vi "Analogico_digital_Controlador.vi"() -> ()   [LabVIEW 2015]
panel:
  out "Puntos 2":sgl[](array[numeric])
  out "Puntos":sgl[](array[numeric])
  in  "Boolean":bool
  out "Waveform Graph 3":sgl[](graph)
  out "Waveform Graph 2":sgl[](graph)
  out "Número de ejes detectados":i32
  out "Waveform Graph":sgl[](graph)
  in  "file (use dialog)":path
  out "deleted portion":sgl[](array[numeric])
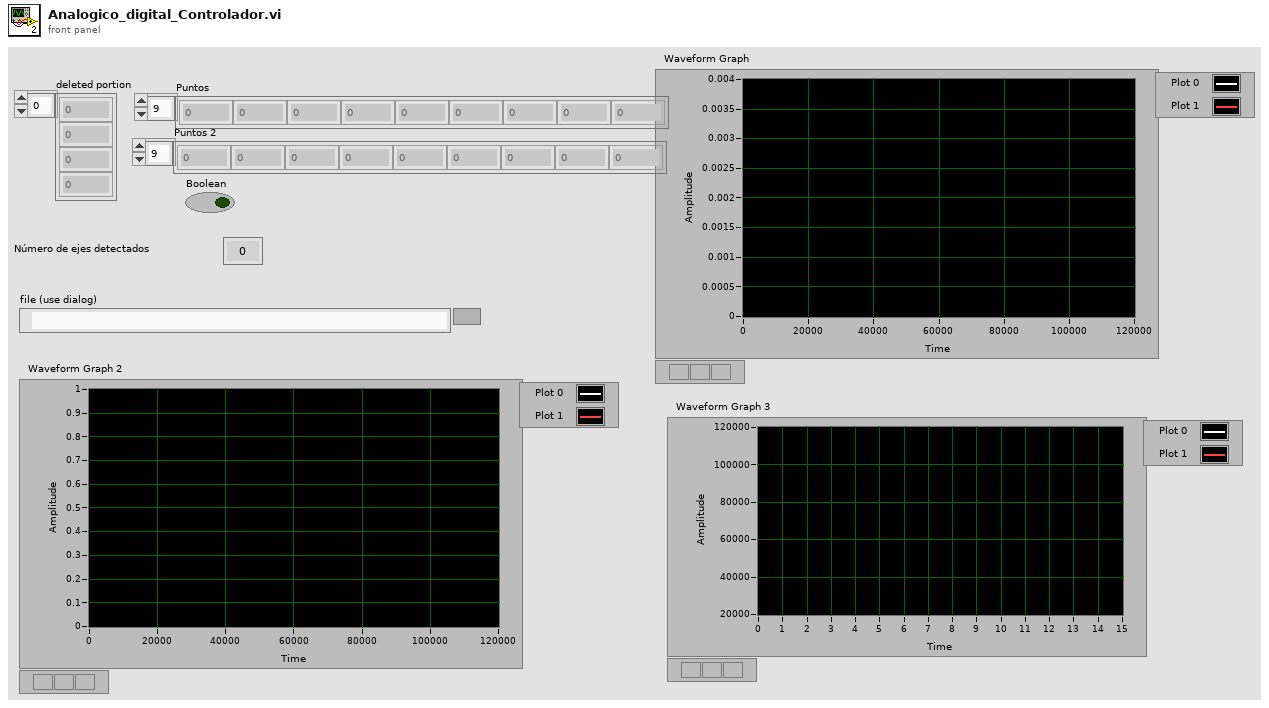
[diagram p1: front panel]
types:
  T1 = enum16{"big-endian, network order", "native, host order", "little-endian"}
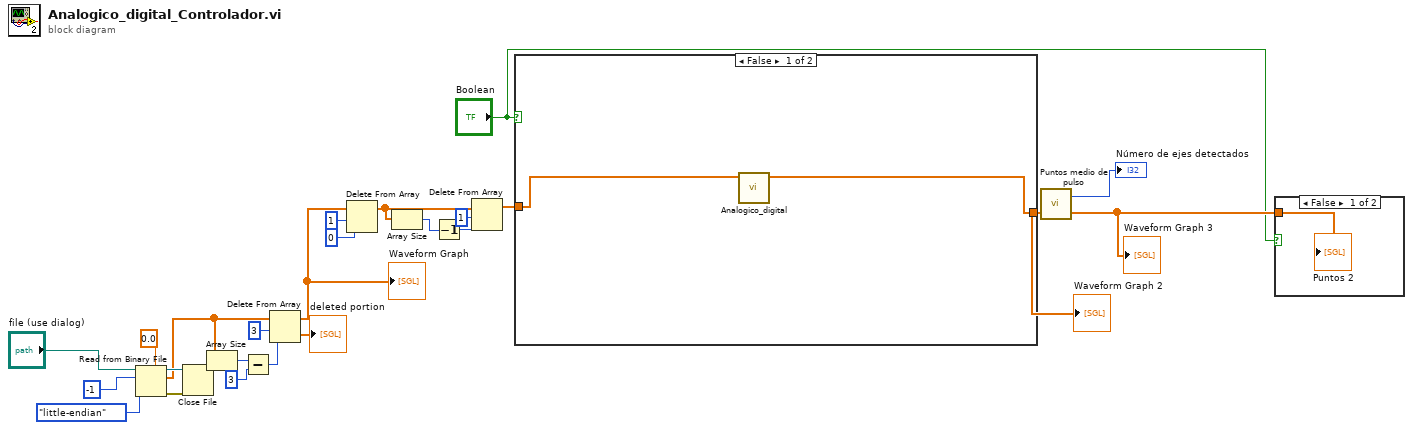
[diagram p0: block diagram]
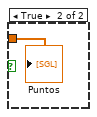
[diagram p2: hidden frame]
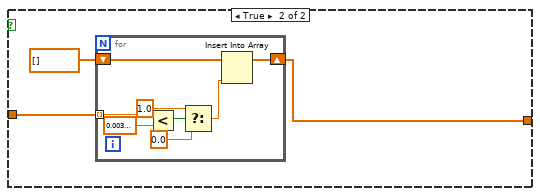
[diagram p3: hidden frame]
diagram:
  n1 = Read from Binary File(5:sgl 0.0, 9:T1."little-endian" ("byte order (0:big-endian, network order)"), 10:-1 ("count (1)"), 11:"file (use dialog)") -> (0:w23:errorcluster, 2:w16:sgl[], 3:w24:refnum<file>)  [unwired: 1 in, 2 out]
  n2 = Close File(refnum=w24, error in=w23) -> ()  [unwired: 2 out]
  n3 = Array Size(array=w16) -> (size(s)=w20:i32)
  n4 = Subtract(x=w20, y=3 ("length")) -> (x-y=w18:i32)
  n5 = Delete From Array(array=w16, length=3, index=w18) -> (deleted portion=→"deleted portion":sgl[], array with subset deleted=w12:sgl[])
  "Waveform Graph" <- w12
  n6 = Delete From Array(array=w12, length=1, index=0) -> (array with subset deleted=w9:sgl[])  [unwired: 1 out]
  n7 = Array Size(array=w9) -> (size(s)=w7:i32)
  n8 = Decrement(x=w7) -> (x-1=w8:i32)
  n9 = Delete From Array(array=w9, length=1, index=w8) -> (array with subset deleted=w3:sgl[])  [unwired: 1 out]
  n10 = case shown="False" "Boolean" {
    tunnel: [w25 w28] -> w5
    tunnel: w3 -> [w26 w27]
    frame False {
      n11 = call "Analogico_digital.vi"("Array"=w26) -> ("array w/ subset deleted"=w25:sgl[])  [unwired: 10 in]
    }
    frame True {
      n12 = for {
        tunnel: w27 -> [w37] mode=indexing
        shift-right: [w30] -> w28
        shift-left: sgl[] [] ("array w/ subset deleted") -> [w31]
        n13 = Less?(x=w37, y=sgl 0.003) -> (x < y?=w35:bool)
        n14 = Select(t=1.0, s=w35, f=0.0) -> (s? t:f=w32:dbl)
        n15 = Insert Into Array(array=w31, new element=w32) -> (w30:sgl[])  [unwired: 1 in]
      }
    }
  }
  "Waveform Graph 2" <- w5
  n16 = call "Puntos medio de pulso.vi"("DI Inductivo"=w5) -> ("Puntos"=w2:sgl[], "Número de ejes"=→"Número de ejes detectados":i32)  [unwired: 1 in]
  "Waveform Graph 3" <- w2
  n17 = case shown="False" "Boolean" {
    tunnel: w2 -> [w38 w39]
    frame False {
      "Puntos 2" <- w38
    }
    frame True {
      "Puntos" <- w39
    }
  }
